vi "generatedatafilename.vi"(1 "timestamp":timestamp, 2 "filename prefix in":string) -> (0 "full-filename":string="20140304-163843-")   [LabVIEW 2015]
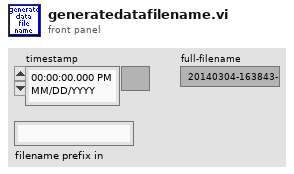
[diagram p1: front panel]
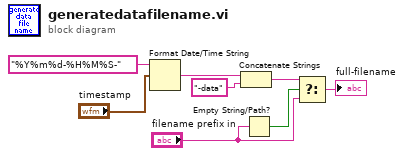
[diagram p0: block diagram]
diagram:
  n1 = Format Date/Time String(time format string (%c)="%Y%m%d-%H%M%S-", seconds (now)="timestamp") -> (date/time string=w7:string)  [unwired: 1 in]
  n2 = Concatenate Strings(w7, "-data" ("t")) -> (w3:string)
  n3 = Empty String/Path?(string/path="filename prefix in") -> (empty?=w5:bool)
  n4 = Select(t=w3, s=w5, f="filename prefix in") -> (s? t:f=→"full-filename":string)
